vi "neslabInit.vi"(3 "error in (no error)":errorcluster, 5 "COM Port":refnum<visa-resource-name>="COM12") -> (0 "error out":errorcluster, 1 "Numeric Return":dbl format="%.2f", 2 "COM Port Out":refnum<visa-resource-name>)   [LabVIEW 2010]
uses:
  <vilib>/Instr/_visa.llb/VISA Configure Serial Port (Instr).vi
panel:
  out "Return Dialog":string
  out "Serial Read":string
  out "byte array\n(out)":string[](array[string])
  in  "byte array\n(in)":string[](array[string])=["CA", "00", "01", "00", "00", "FE"]
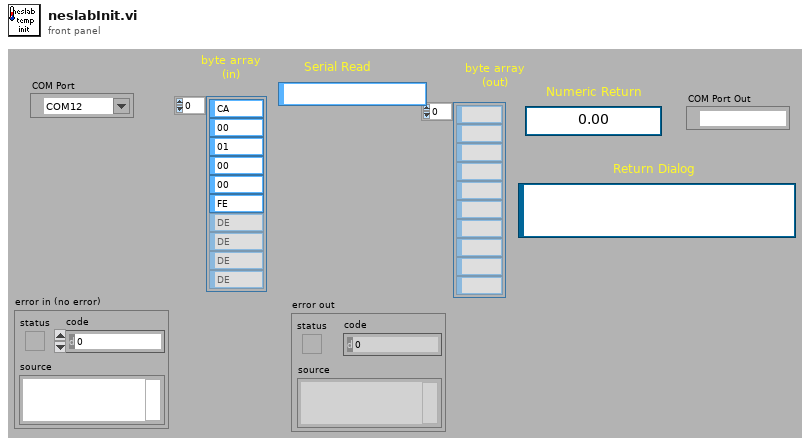
[diagram p1: front panel]
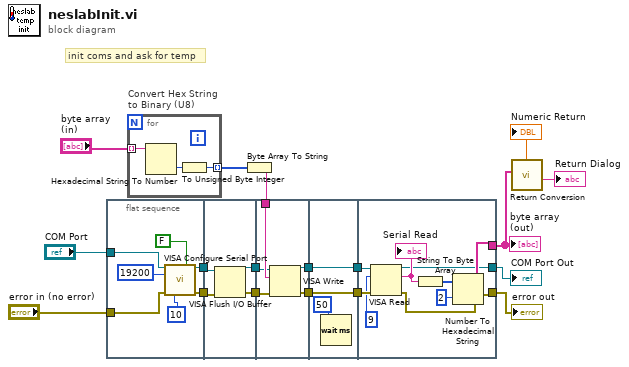
[diagram p0: block diagram]
diagram:
  # "init coms and ask for temp"
  # "Convert Hex String \nto Binary (U8)"
  n1 = flat-sequence {
    tunnel: [w23] -> w16
    tunnel: [w22] -> w15
    tunnel: "error in (no error)" -> [w20]
    tunnel: "COM Port" -> [w19]
    tunnel: w16 -> [w28]
    tunnel: w15 -> [w27]
    tunnel: [w29] -> w9
    tunnel: [w26] -> w8
    tunnel: w12 -> [w34]
    tunnel: w9 -> [w33]
    tunnel: w8 -> [w30]
    tunnel: [w32] -> w7
    tunnel: [w31] -> w6
    tunnel: [w37] -> w14
    tunnel: [w36] -> w13
    tunnel: w7 -> [w37]
    tunnel: w6 -> [w36]
    tunnel: [w42] -> w11
    tunnel: [w41] -> w10
    tunnel: w14 -> [w40]
    tunnel: w13 -> [w39]
    tunnel: [w43] -> w3
    frame #0 {
      n2 = call-poly "VISA Configure Serial Port"("VISA resource name"=w19, "Enable Termination\nChar (T)"=FALSE, "baud rate (9600)"=u32 19200 ("Baud Rate"), "error in (no error)"=w20, "stop bits (10: 1 bit)"=10) -> ("VISA resource name out"=w23:refnum<visa-resource-name>, "error out"=w22:errorcluster)  [unwired: 9 in]
    }
    frame #1 {
      n3 = VISA Flush I/O Buffer(VISA resource name=w28, error in (no error)=w27) -> (VISA resource name out=w29:refnum<visa-resource-name>, error out=w26:errorcluster)  [unwired: 1 in]
    }
    frame #2 {
      n4 = VISA Write(VISA resource name=w33, write buffer=w34, error in (no error)=w30) -> (VISA resource name out=w32:refnum<visa-resource-name>, error out=w31:errorcluster)  [unwired: 1 out]
    }
    frame #3 {
      n5 = Wait (ms)(milliseconds to wait=50) -> ()  [unwired: 1 out]
    }
    frame #4 {
      n6 = VISA Read(VISA resource name=w40, byte count=9, error in (no error)=w39) -> (VISA resource name out=w41:refnum<visa-resource-name>, read buffer=w44:string, error out=w42:errorcluster)  [unwired: 1 out]
      "Serial Read" <- w44
      n7 = String To Byte Array(string=w44) -> (unsigned byte array=w46:u8[])
      n8 = Number To Hexadecimal String(1:2, 2:w46) -> (0:w43:string[])
    }
  }
  n9 = for {
    tunnel: "byte array\n(in)" -> [w49] mode=indexing
    tunnel: [w47] -> w18 mode=indexing
    n10 = Hexadecimal String To Number(string=w49) -> (number=w48:u32)  [unwired: 2 in, 1 out]
    n11 = To Unsigned Byte Integer(number=w48) -> (unsigned 8bit integer=w47:u8)
  }
  n12 = Byte Array To String(unsigned byte array=w18) -> (string=w12:string)
  n13 = call "Return Conversion.VI"("Input Array"=w3) -> ("Numeric\nReading\nValue"=→"Numeric Return":dbl, "Reading String\nwith Descriptor"=→"Return Dialog":string)  [unwired: 7 in]
  "COM Port Out" <- w10
  "error out" <- w11
  "byte array\n(out)" <- w3
